vi "Actor Core.vi"(8 "error in":errorcluster, 11 "Nested in":refnum<class "Calling Actor.lvclass">) -> (0 "error out":errorcluster, 3 "Actor out":refnum<class "Actor.lvclass">)   [LabVIEW 2019, in "Calling Actor.lvlib" / "Calling Actor.lvclass"]
doc: "(<B>Filename</B>: Actor Framework.lvlib:Actor.lvclass:Actor Core.vi)\n\nReceives messages to the actor, reacts to them, and initiates any error handling that may shut the actor down.\n\nDescendant classes may override this VI to append parallel tasks for the actor to complete while it handles messages. Overrides use the Call Parent Method node."
uses:
  Calling Actor.lvclass
  C:/Program Files (x86)/National Instruments/LabVIEW 2019/vi.lib/ActorFramework/Actor/Actor.lvclass
  <vilib>/ActorFramework/Actor/Actor.lvclass
  Calling Actor.lvclass/Calling Actor.ctl
  <vilib>/ActorFramework/Actor/Actor.lvclass/Actor.ctl
  <vilib>/ActorFramework/Message Enqueuer/Message Enqueuer.lvclass/Message Enqueuer.ctl
  Calling Actor Messages/Send Nested Actor Message Msg/Send Nested Actor Message Msg.lvclass/Send Nested Actor Message Msg.ctl
  <vilib>/ActorFramework/Message Enqueuer/Init from Existing Queue.vi
  <vilib>/ActorFramework/Message Enqueuer/Enqueue.vi
  Calling Actor Messages/Launch Nested Actor Msg/Launch Nested Actor Msg.lvclass
  C:/Program Files (x86)/National Instruments/LabVIEW 2019/vi.lib/ActorFramework/Message/Message.lvclass
  Calling Actor Messages/Send Nested Actor Message Msg/Send Nested Actor Message Msg.lvclass
  <vilib>/ActorFramework/Stop Msg/Stop Msg.lvclass
  <vilib>/ActorFramework/Message Priority Queue/Priority Enqueue.vi
  <vilib>/ActorFramework/Message Enqueuer/Message Enqueuer.lvclass
panel:
  in  "Launch New Actor":bool
  in  "Nested Actor":string(combo)
  in  "Send Message":bool
  in  "Message":string
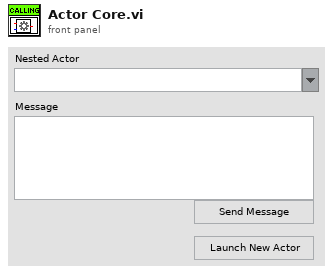
[diagram p1: front panel]
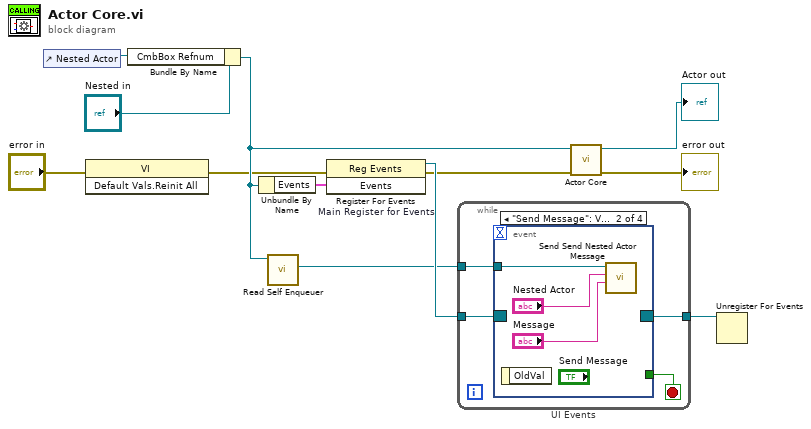
[diagram p0: block diagram]
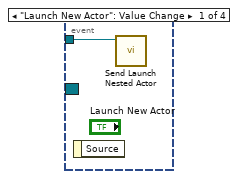
[diagram p2: hidden frame]
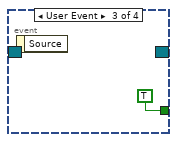
[diagram p3: hidden frame]
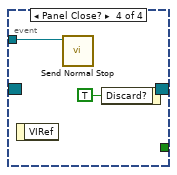
[diagram p4: hidden frame]
diagram:
  n1 = control-ref of="Nested Actor"() -> (w3:refnum<vi>)
  n2 = invoke class="VI" method="Default Vals.Reinit All"(error in="error in") -> (error out=w2:errorcluster)  [unwired: 2 in, 2 out]
  n3 = Bundle By Name(cluster="Nested in", "CmbBox Refnum"=w3) -> (w4:refnum<class "Calling Actor.lvclass">)
  n4 = Unbundle By Name(w4) -> ("Events"=w9:cluster{"Stop":refnum<user-event>})
  n5 = call <vilib>:"Read Self Enqueuer.vi"("Actor"=w4) -> ("Self Enqueuer"=w7:refnum<class "Message Enqueuer.lvclass">)  [unwired: 10 in]
  n6 = register-events "Main Register for Events"(error in=w2, w9) -> (reference out=w10:refnum<event-registration>, error out=w6:errorcluster)  [unwired: 1 in]
  n7 = while {
    tunnel: w10 -> [w16]
    tunnel: [w14] -> w8
    tunnel: w7 -> [w13]
    stop <- w15 stop-if-true
    n8 = event "UI Events" shown="[1] \"Send Message\": Value Change" {
      selector: w16 -> [_ _ _ _]
      dyn-events: [_ _ _ _] -> w14
      timeout: _ -> [_ _ _ _]
      tunnel: [_ _ TRUE _] -> w15
      tunnel: w13 -> [w17 w20 _ w22]
      event "Launch New Actor": Value Change {
        n9 = event-data() -> ()  [unwired: 1 in, 1 out]
        n10 = call "Send Launch Nested Actor.vi"("Message Enqueuer"=w17) -> ()  [unwired: 9 in, 2 out]
      }
      event "Send Message": Value Change {
        n11 = event-data() -> ()  [unwired: 1 in, 1 out]
        n12 = call "Send Send Nested Actor Message.vi"("Message"="Message", "Actor Name"="Nested Actor", "Message Enqueuer"=w20) -> ()  [unwired: 7 in, 2 out]
      }
      event User Event {
        n13 = event-data() -> ()  [unwired: 1 in, 1 out]
      }
      event Panel Close? {
        n14 = event-data() -> ()  [unwired: 1 in, 1 out]
        n15 = call <vilib>:"Send Normal Stop.vi"("Message Enqueuer"=w22) -> ()  [unwired: 10 in, 1 out]
        n16 = event-data("Discard?"=TRUE) -> ()  [unwired: 1 in, 1 out]
      }
    }
  }
  n17 = call-parent "Actor Core.vi"("error in"=w6, "Actor in"=w4) -> ("error out"=→"error out":errorcluster, "Actor out"=→"Actor out":refnum<class "Actor.lvclass">)  [unwired: 8 in]
  n18 = Unregister For Events(event registration refnum=w8) -> ()  [unwired: 1 in, 1 out]
